vi "Read AH2700A (SubVI).vi"(8 "error in (no error)":errorcluster, 11 "VISA Refnum in":refnum<visa-resource-name>) -> (0 "error out":errorcluster, 1 "Loss":dbl format="%#_10f", 2 "Capacitance":dbl format="%#_10f", 3 "VISA Refnum out":refnum<visa-resource-name>, 4 "Units 2":i32(ring) items=["", "nanosiemens", "dissipation factor", "kilohms", "gigohms", "loss vector (jpF)"], 5 "Voltage":dbl, 7 "Frequency":dbl)   [LabVIEW 2025]
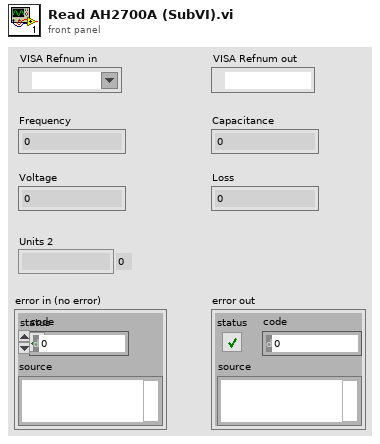
[diagram p1: front panel]
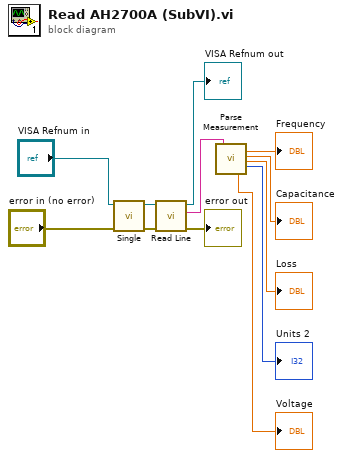
[diagram p0: block diagram]
diagram:
  n1 = call "Single.vi"("error in"="error in (no error)", "VISA resource name"="VISA Refnum in") -> ("error out"=w9:errorcluster, "VISA resource name out"=w8:refnum<visa-resource-name>)  [unwired: 8 in]
  n2 = call "Read Line.vi"("error in"=w9, "VISA resource name"=w8) -> ("error out"=→"error out":errorcluster, "Message"=w5:string, "VISA resource name out"=→"VISA Refnum out":refnum<visa-resource-name>)  [unwired: 5 in, 2 out]
  n3 = call "Parse Measurement.vi"("Measurement Line"=w5) -> ("Voltage"=→"Voltage":dbl, "Frequency"=→"Frequency":dbl, "Capacitance"=→"Capacitance":dbl, "Loss"=→"Loss":dbl, "Units"=→"Units 2":i32)  [unwired: 10 in, 4 out]
